vi "CRUD Read Example.vi"() -> ()   [LabVIEW 2020, in "ORM_Examples.lvlib"]
doc: "Returns one result from the query for which \"playerNum\" is specified. Since playerNum is the primary key for the corresponding table, only 1 or 0 results may be returned. The returned data set is mapped to the private data of the bbPlayers class. Note that BB Players Map class is also needed."
uses:
  ORM_Examples.lvlib
  BB Players/bbPlayers.lvclass
  BB Players Map/BB Players Map.lvclass
  C:/Program Files/National Instruments/LabVIEW 2020/vi.lib/Viviota/shared/ORM.lvlibp/ORM/TypeMap/TypeMap.lvclass
  a3bda483-7bd3-497e-924e-0676829bf577.vi
  a3bda483-7bd3-497e-924e-0676829bf577.vi/ce8babb2-619c-4b95-b634-e027cd54a13e.vi
  a3bda483-7bd3-497e-924e-0676829bf577.vi/383c36e0-7191-4c70-923d-4cc1411f3794.vi
  a3bda483-7bd3-497e-924e-0676829bf577.vi/dcffdf9a-60b2-440f-af14-9d618c05381d.vi
  <vilib>/Viviota/shared/ORM_ADONet.lvlibp/ADOMapper/ADOMapper.lvclass
  C:/Program Files/National Instruments/LabVIEW 2020/vi.lib/Viviota/shared/ORM.lvlibp/ORM/SqlMapper/SqlMapper.lvclass
  <vilib>/Viviota/shared/ORM.lvlibp/ORM/TypeMap/Write Autokey.vi
  <vilib>/Viviota/shared/ORM.lvlibp/ORM/TypeMap/Write Table Name.vi
  DbConnections/SqliteConnection/Sqlite Connect.vi
  <vilib>/Utility/error.llb/Error Cluster From Error Code.vi
  <vilib>/Viviota/shared/ORM.lvlibp/ORM/TypeMap/Read TypeMap.vi
  <vilib>/Viviota/shared/ORM.lvlibp/ORM/SqlMapper/End Transaction.vi
  <vilib>/Viviota/shared/ORM.lvlibp/ORM/TypeMap/TypeMap.lvclass
  ORM_API/ORM_API.lvlib
  <vilib>/Viviota/shared/ORM_ADONet.lvlibp
  DbConnections/SqliteConnection/DBC.lvclass
  C:/Program Files/National Instruments/LabVIEW 2020/vi.lib/Viviota/shared/ORM_ADONet.lvlibp/ADOMapper/ADOMapper.lvclass
panel:
  out "pNum":i32
  out "pName":string
  out "pGames":i32
  out "pAverage":dbl
  out "pAvailable":bool
  in  "playerNum":i32
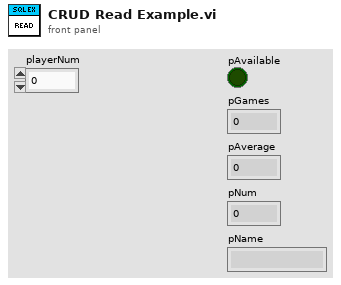
[diagram p1: front panel]
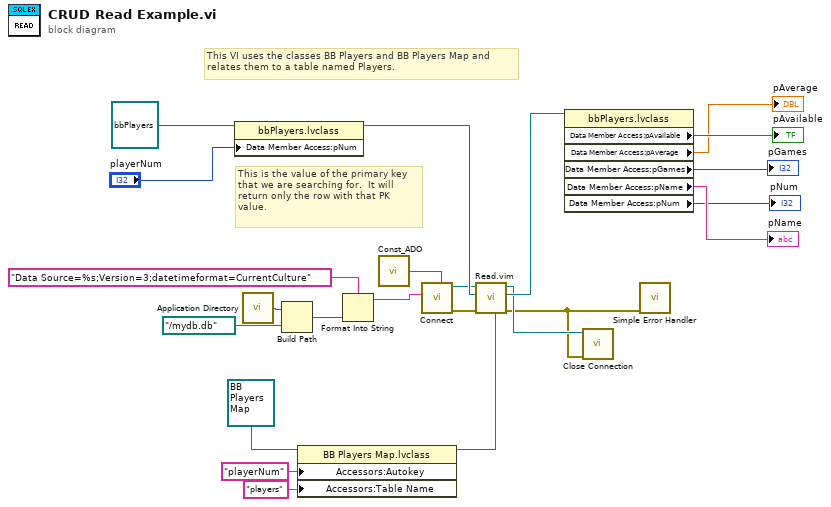
[diagram p0: block diagram]
diagram:
  # "This VI uses the classes BB Players and BB Players Map and \nrelates them to a table named Players."
  # "This is the value of the primary key\nthat we are searching for.  It will\nreturn only the row with that PK\nvalue."
  n1 = property class="bbPlayers.lvclass"(reference=refnum<class "bbPlayers.lvclass"> refnum ("bbPlayers.lvclass"), "Data Member Access:pNum"="playerNum") -> (reference out=w21:refnum<class "bbPlayers.lvclass">)  [unwired: 1 in, 1 out]
  n2 = call <vilib>:"Application Directory.vi"() -> ("Application Directory"=w9:path)
  n3 = Build Path(base path=w9, name or relative path=path "../mydb.db" ("file out")) -> (appended path=w10:path)
  n4 = property class="BB Players Map.lvclass"(reference=refnum<class "BB Players Map.lvclass"> refnum ("BB Players Map.lvclass"), "Accessors:Autokey"="playerNum" ("Autokey"), "Accessors:Table Name"="players" ("Table Name")) -> (reference out=w17:refnum<class "BB Players Map.lvclass">)  [unwired: 1 in, 1 out]
  n5 = Format Into String(format string="Data Source=%s;Version=3;datetimeformat=CurrentCulture" ("connectionStringName"), w10) -> (resulting string=w5:string)  [unwired: 2 in, 1 out]
  n6 = call <vilib>:"Const_ADO.vi"() -> ("ADOMapper"=w6:refnum<class "ADOMapper.lvclass">)
  n7 = call-poly "Connect.vi"("SqlMapper Type"=w6, "Connection String"=w5) -> ("error out"=w3:errorcluster, "SqlMapper out"=w4:refnum<class "ADOMapper.lvclass">)  [unwired: 8 in]
  n8 = call "Read.vim"("TypeMap in"=w17, "error in (no error)"=w3, "object in"=w21, "SqlMapper in"=w4) -> ("error out"=w1:errorcluster, "object out"=w16:refnum<class "bbPlayers.lvclass">, "SqlMapper out"=w2:refnum<class "SqlMapper.lvclass">)  [unwired: 4 in, 1 out]
  n9 = property class="bbPlayers.lvclass"(reference=w16) -> ("Data Member Access:pAvailable"=→"pAvailable":bool, "Data Member Access:pAverage"=→"pAverage":dbl, "Data Member Access:pGames"=→"pGames":i32, "Data Member Access:pName"=→"pName":string, "Data Member Access:pNum"=→"pNum":i32)  [unwired: 1 in, 2 out]
  n10 = call "Close Connection.vi"("Error In"=w1, "SqlMapper"=w2) -> ()  [unwired: 9 in, 1 out]
  n11 = call <vilib>:"Simple Error Handler.vi"("error in (no error)"=w1) -> ()  [unwired: 4 in, 5 out]
